vi "Cache.Write.vi"(7 "Idx":i32, 8 "error in (no error)":errorcluster, 10 "Results":T4 {"Values" format="%.3f"}, 11 "Data in":T1) -> (0 "error out":errorcluster, 3 "Data out":T1)   [LabVIEW 2016]
uses:
  Cache.ProductComponent.Data.ctl
  Tools/EventLog/EventLog.EventSource.ctl
  Tools/Translator/Translator.Message.ctl
  Cache.Status.Fglb.Action.ctl
  Tools/EventLog/EventLog.New(array).vi
  Drivers/PLC/LowLevel/PLC.DataBlock.PLCvalues.ctl
  Cache.Data.Status.ctl
  Cache.Data.Sets.ctl
  Cache.Data.ctl
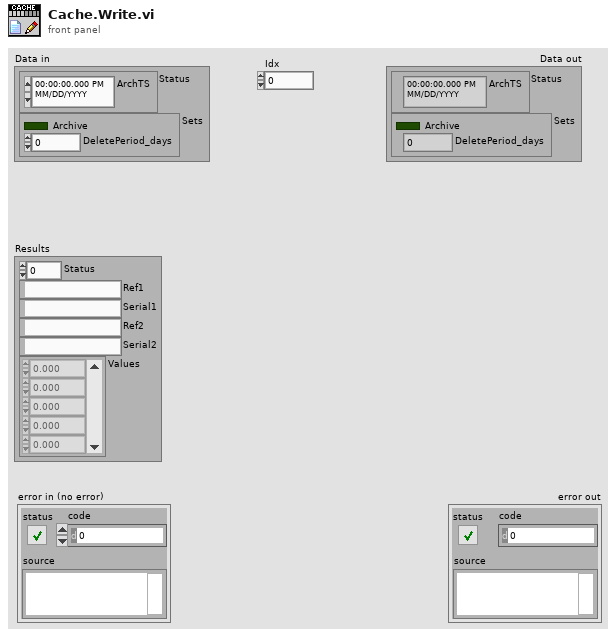
[diagram p1: front panel]
types:
  T1 = typedef "Cache.Data.ctl" = cluster{"Status":T2, "Sets":T3}
  T2 = typedef "Cache.Data.Status.ctl" = cluster{"ArchTS":timestamp}
  T3 = typedef "Cache.Data.Sets.ctl" = cluster{"Archive":bool, "DeletePeriod_days":dbl}
  T4 = typedef "PLC.DataBlock.PLCvalues.ctl" = cluster{"Status":u8, "Ref1":string, "Serial1":string, "Ref2":string, "Serial2":string, "Values":sgl[]}
  T5 = typedef "Cache.Status.Fglb.Action.ctl" = enum16{"init", "Changeover", "CheckStatus", "NewData", "get"}
  T6 = typedef "Translator.Message.ctl" = enum16{"-", "Event confirmed", "Log out", "Log in", "Shutdown", "Cancel", "Start", "Continue", "Stop", "On", "Off", "OK", "NOK", "NOK %s", "This", "Prev", "Home", "Work", "In progress...", "Missing", "Empty", "Hardware failure", "Initial", "Error %d >> %s", "Error %d >> %s >> %s", "Starting %s", "Quitting %s", "Configured", "Initializing", "Quitting", "Loading", "Running %s", "Stopped", "Summary", "Do you want to continue?", "Do you want to exit?", "Log out?", "System", "All", "IDLE", "Translating...%s", "Not found", "Alarm %s", "Run", "Skip", "Abort", "Repeat", "Please wait...", "Database disconnected", "Login to database successful", "Login to database failed: %d; %s", "Get process step data for %s", "Changeover off", "Changeover into %s", "Product %s | %s found in cache with status %d at previous station", "Product %s | %s found in database with status %d at previous station", "Product %s | %s not found in cache at previous station", "Product %s | %s not found in database at previous station", "Product %s | %s found in cache with status %d at this station (%d repetion)", "Product %s | %s found in database with status %d at this station (%d repetition)", "Product %s | %s not found in cache at this station", "Product %s | %s not found in database at this station", "Product %s | %s found in cache for component %s | %s", "Product %s | %s found in database for component %s | %s", "Product not found in cache for component %s | %s", "Product not found in database for component %s | %s", "Product %s | %s connected with component %s | %s (cache)", "Product %s | %s connected with component %s | %s (database)", "New data for %s | %s (cache)", "New data for %s | %s (database)", "File %s moved (cache)", "Msg %d >> %s", "PLC LifeBit Failure", "Reconnecting DB", "Reconnecting PLC"}
  T7 = typedef "EventLog.EventSource.ctl" = enum16{"All", "Gui", "Cache", "PLC1", "PLC2", "PLC3", "DB", "DB01", "DB02", "DB03", "DB04", "DB05", "DB06", "DB07", "DB08", "DB09", "DB10", "DB11", "DB12", "DB13", "DB14", "DB15", "DB16"}
  T8 = typedef "Cache.ProductComponent.Data.ctl" = cluster{"Time":timestamp, "Station":string, "Ref1":string, "Serial1":string, "Ref2":string, "Serial2":string}
  T9 = typedef "Cache.TestSteps.Fglb.ResultData.ctl" = cluster{"Ref":string, "Serial":string, "Pr":T10, "PSr":T11, "TSr":cluster{"TSr":T12, "TVr":T13[]}[]}
  T10 = typedef "ProdaNG.ProcessResult.ctl" = cluster{"c_id":string, "productId":string, "processId":i32, "statusId":i32, "startTime":string, "endTime":string}
  T11 = typedef "ProdaNG.ProcessStepResult.ctl" = cluster{"c_id":string, "processResultId":string, "processStepId":i32, "statusId":i32, "operatorId":i32, "startTime":string, "endTime":string}
  T12 = typedef "ProdaNG.TestStepResult.ctl" = cluster{"c_id":string, "processStepResultId":string, "testStepId":i32, "statusId":i32}
  T13 = typedef "ProdaNG.TestValueResult.ctl" = cluster{"c_id":string, "testStepResultId":string, "testValueId":i32, "result":dbl, "statusId":i32, "contentId":string}
  T14 = typedef "Cache.TestSteps.Fglb.TestData.ctl" = cluster{"Ref":string, "Desc":string, "P":T15, "PS":T16, "PP":T17[], "TS":cluster{"TS":T18, "TV":T19[], "TP":T20[]}[], "Units":T21[]}
  T15 = typedef "ProdaNG.Process.ctl" = cluster{"i_id":i32, "productionLineId":i32, "releaseId":i32, "contentId":string, "previewId":string, "mdReason":string, "mdUser":string, "mdTime":string, "description":string}
  T16 = typedef "ProdaNG.ProcessStep.ctl" = cluster{"i_id":i32, "processId":i32, "systemId":i32, "releaseId":i32, "processSequence":i32, "limitYellow":dbl, "limitRed":dbl, "mdReason":string, "mdUser":string, "mdTime":string, "filename":string, "transfer":string, "description":string}
  T17 = typedef "ProdaNG.ProcessStepParam.ctl" = cluster{"i_id":i32, "processStepId":i32, "unitId":i32, "contentId":string, "previewId":string, "value":dbl, "valueText":string, "paramSequence":i32, "history":i32, "mdReason":string, "mdUser":string, "mdTime":string, "description":string}
  T18 = typedef "ProdaNG.TestStep.ctl" = cluster{"i_id":i32, "processStepId":i32, "testSequence":i32, "testOrder":i32, "mdReason":string, "mdUser":string, "mdTime":string, "description":string}
  T19 = typedef "ProdaNG.TestValue.ctl" = cluster{"i_id":i32, "testStepId":i32, "releaseId":i32, "unitId":i32, "contentId":string, "previewId":string, "maximum":dbl, "minimum":dbl, "valueText":string, "testValueSequence":i32, "history":i32, "mdReason":string, "mdUser":string, "mdTime":string, "description":string}
  T20 = typedef "ProdaNG.TestStepParam.ctl" = cluster{"i_id":i32, "testStepId":i32, "unitId":i32, "contentId":string, "previewId":string, "value":dbl, "valueText":string, "paramSequence":i32, "history":i32, "mdReason":string, "mdUser":string, "mdTime":string, "description":string}
  T21 = typedef "ProdaNG.Unit.ctl" = cluster{"i_id":i32, "name":string, "mdReason":string, "mdUser":string, "mdTime":string, "description":string}
  T22 = typedef "Database.Data.Sets.ctl" = cluster{"Enable":bool, "ConnString":string, "SystemName":string, "Process.Begin":bool, "Process.End":bool}
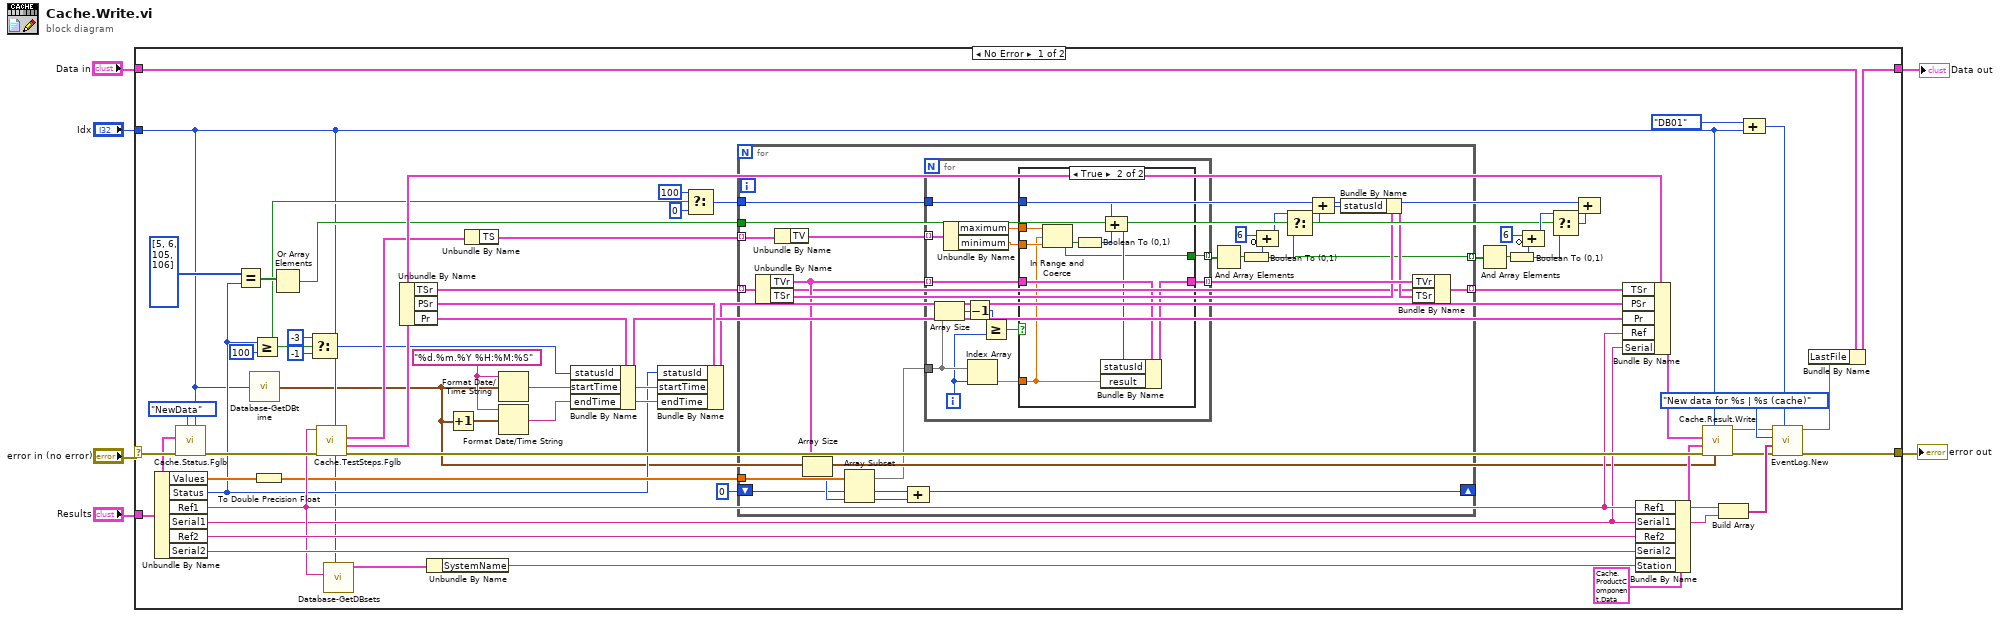
[diagram p0: block diagram]
diagram:
  n1 = case shown="No Error" "error in (no error)" {
    selector: "error in (no error)" -> [w44 w112]
    tunnel: [w10 w112] -> w3
    tunnel: "Results" -> [w41 _]
    tunnel: "Idx" -> [w12 _]
    tunnel: "Data in" -> [w9 w111]
    tunnel: [w8 w111] -> w1
    frame No Error {
      w61 = "%d.%m.%Y %H:%M:%S" ("time format string (%c)")
      n2 = Unbundle By Name(w41) -> ("Values"=w65:sgl[], "Status"=w13:u8, "Ref1"=w38:string, "Serial1"=w37:string, "Ref2"=w52:string, "Serial2"=w53:string)
      n3 = call "Cache.Status.Fglb.vi"("SystemIdx"=w12, "Action (get)"=Cache.Status.Fglb.Action."NewData", "error in (no error)"=w44, "NewData"=w41) -> ("error out"=w43:errorcluster)  [unwired: 6 in, 1 out]
      n4 = Equal?(x=u8[] [5, 6, 105, 106], y=w13) -> (x = y?=w29:bool[])
      n5 = call "Database-GetDBtime.vi"("Idx"=w12) -> ("DbTime"=w11:timestamp)
      n6 = Greater Or Equal?(x=w13, y=u8 100) -> (x >= y?=w20:bool)
      n7 = To Double Precision Float(number=w65) -> (double precision float=w31:dbl[])
      n8 = Or Array Elements(Boolean array=w29) -> (logical OR=w16:bool)
      n9 = Select(t=-3 ("statusId"), s=w20, f=-1 ("statusId")) -> (s? t:f=w18:i32)
      n10 = call "Cache.TestSteps.Fglb.vi"("SystemIdx"=w12, "error in (no error)"=w43, "Variant"=w38) -> ("error out"=w55:errorcluster, "Result out"=w57:T9, "Test out"=w33:T14)  [unwired: 5 in, 1 out]
      n11 = call "Database-GetDBsets.vi"("Idx"=w12, "Variant"=w38) -> ("Sets"=w39:T22)  [unwired: 5 in, 4 out]
      n12 = Unbundle By Name(w57) -> ("TSr"=w64:cluster{"TSr":T12, "TVr":T13[]}[], "PSr"=w63:T11, "Pr"=w17:T10)
      n13 = Unbundle By Name(w39) -> ("SystemName"=w34:string)
      n14 = Increment(x=w11) -> (x+1=w60:timestamp)
      n15 = Unbundle By Name(w33) -> ("TS"=w32:cluster{"TS":T18, "TV":T19[], "TP":T20[]}[])
      n16 = Format Date/Time String(time format string (%c)=w61, seconds (now)=w11) -> (date/time string=w59:string)  [unwired: 1 in]
      n17 = Format Date/Time String(time format string (%c)=w61, seconds (now)=w60) -> (date/time string=w58:string)  [unwired: 1 in]
      n18 = Bundle By Name(cluster=w17, "statusId"=w18, "startTime"=w59, "endTime"=w58) -> (w15:T10)
      n19 = Bundle By Name(cluster=w63, "statusId"=w13, "startTime"=w59, "endTime"=w58) -> (w14:T11)
      n20 = Select(t=100 ("0, 1"), s=w20, f=0 ("0, 1")) -> (s? t:f=w19:i32)
      n21 = for {
        tunnel: w31 -> [w84]
        tunnel: w64 -> [w66] mode=indexing
        tunnel: [w85] -> w56 mode=indexing
        shift-right: [w79] -> _
        shift-left: 0 -> [w81]
        tunnel: w32 -> [w76] mode=indexing
        tunnel: w19 -> [w67]
        tunnel: w16 -> [w74]
        tunnel: [w68] -> w23 mode=indexing
        n22 = Unbundle By Name(w66) -> ("TVr"=w83:T13[], "TSr"=w86:T12)
        n23 = Unbundle By Name(w76) -> ("TV"=w77:T19[])
        n24 = Array Size(array=w83) -> (size(s)=w82:i32)
        n25 = Array Subset(array=w84, index=w81, length=w82) -> (w80:dbl[])
        n26 = Compound Arithmetic op=ADD(w81, w82) -> (w79:i32)
        n27 = for "results" {
          tunnel: w80 -> [w95]
          tunnel: w83 -> [w100] mode=indexing
          tunnel: [w99] -> w87 mode=indexing
          tunnel: w77 -> [w93] mode=indexing
          tunnel: w67 -> [w89]
          tunnel: [w88] -> w75 mode=indexing
          i -> [w94]
          n28 = Array Size(array=w95) -> (size(s)=w96:i32)
          n29 = Unbundle By Name(w93) -> ("maximum"=w92:dbl, "minimum"=w91:dbl)
          n30 = Decrement(x=w96) -> (x-1=w90:i32)
          n31 = Index Array(array=w95, index=w94) -> (element=w98:dbl)
          n32 = Greater Or Equal?(x=w90, y=w94) -> (x >= y?=w97:bool)
          n33 = case shown="True" w97 {
            tunnel: w100 -> [w101 w110]
            tunnel: [w101 w109] -> w99
            tunnel: w98 -> [_ w106]
            tunnel: w92 -> [_ w108]
            tunnel: w91 -> [_ w107]
            tunnel: w89 -> [_ w102]
            tunnel: [_ w103] -> w88
            frame False {
            }
            frame True {
              n34 = In Range and Coerce(upper limit=w108, x=w106, lower limit=w107) -> (In Range?=w103:bool)  [unwired: 1 out]
              n35 = Boolean To (0,1)(Boolean=w103) -> (0, 1=w105:i16)
              n36 = Compound Arithmetic op=ADD(w102, w105) -> (w104:i32)
              n37 = Bundle By Name(cluster=w110, "statusId"=w104, "result"=w106) -> (w109:T13)
            }
          }
        }
        n38 = And Array Elements(Boolean array=w75) -> (logical AND=w68:bool)
        n39 = Boolean To (0,1)(Boolean=w68) -> (0, 1=w73:i16)
        n40 = Compound Arithmetic op=ADD(i16 6 ("0, 1"), invert w73) -> (w71:i16)
        n41 = Select(t=w71, s=w74, f=w73) -> (s? t:f=w70:i16)
        n42 = Compound Arithmetic op=unknown(w67, w70) -> (w69:i32)
        n43 = Bundle By Name(cluster=w86, "statusId"=w69) -> (w78:T12)
        n44 = Bundle By Name(cluster=w66, "TVr"=w87, "TSr"=w78) -> (w85:cluster{"TSr":T12, "TVr":T13[]})
      }
      n45 = And Array Elements(Boolean array=w23) -> (logical AND=w24:bool)
      n46 = Boolean To (0,1)(Boolean=w24) -> (0, 1=w25:i16)
      n47 = Compound Arithmetic op=ADD(i16 6 ("0, 1"), invert w25) -> (w27:i16)
      n48 = Select(t=w27, s=w16, f=w25) -> (s? t:f=w28:i16)
      n49 = Compound Arithmetic op=ADD(w19, w28) -> ()  [unwired: 1 out]
      n50 = Bundle By Name(cluster=w57, "TSr"=w56, "PSr"=w14, "Pr"=w15, "Ref"=w38, "Serial"=w37) -> (w40:T9)
      n51 = Bundle By Name(cluster=T8 {"Time"=timestamp(0 s since 1904-01-01), "Station"="", "Ref1"="", "Serial1"="", "Ref2"="", "Serial2"=""} ("ProdComp"), "Ref1"=w38, "Serial1"=w37, "Ref2"=w52, "Serial2"=w53, "Station"=w34) -> (w35:T8)
      n52 = call "Cache.Result.Write.vi"("Time (now)"=w11, "Idx"=w12, "error in (no error)"=w55, "ProdComp"=w35, "Result in"=w40) -> ("error out"=w36:errorcluster, "File"=w7:string)  [unwired: 5 in]
      n53 = Build Array(w38, w37) -> (w45:string[])
      n54 = Compound Arithmetic op=ADD(EventLog.EventSource."DB01" ("Source (All)"), w12) -> (w47:i32)
      n55 = call-poly "EventLog.New.vi"("Source (All)"=w47, "error in (no error)"=w36, "Arguments"=w45, "Message (-)"=Translator.Message."New data for %s | %s (cache)") -> ("error out"=w10:errorcluster)  [unwired: 6 in, 1 out]
      n56 = Bundle By Name(cluster=w9, "LastFile"=w7) -> (w8:T1)
    }
    frame Error {
    }
  }
  "error out" <- w3
  "Data out" <- w1
